vi "insert_block.vi"(8 "error in (no error)":errorcluster, 11 "ImageAssemblerDL090211Frame in":refnum<class "ImageAssemblerDL090211Frame.lvclass">) -> (0 "error out":errorcluster, 3 "ImageAssemblerDL090211Frame out":refnum<class "ImageAssemblerDL090211Frame.lvclass">)   [LabVIEW 2010, in "ImageAssemblerDL090211Frame.lvclass"]
uses:
  ImageAssemblerDL090211Frame.lvclass
  ImageAssemblerDL090211Frame.lvclass/ImageAssemblerDL090211Frame.ctl
  common/classes/Image/Image/Image.lvclass
  common/classes/Image/Image/insert_mode_enum.ctl
  ImagingMode/GenericImagingMode/GenericImagingMode/trigger_enum.ctl
  ImagingMode/GenericImagingMode/GenericImagingMode/GenericImagingMode.lvclass
  common/classes/GenericComponent/GenericComponent/class_data.vi
  ImageAssemblerDL090211Scaffold/ImageAssemblerDL090211Scaffold/ImageAssemblerDL090211Scaffold.lvclass
  common/classes/GenericComponent/GenericComponent/GenericComponent.lvclass
panel:
  out "raw channels":T1[](array[plugin-control])
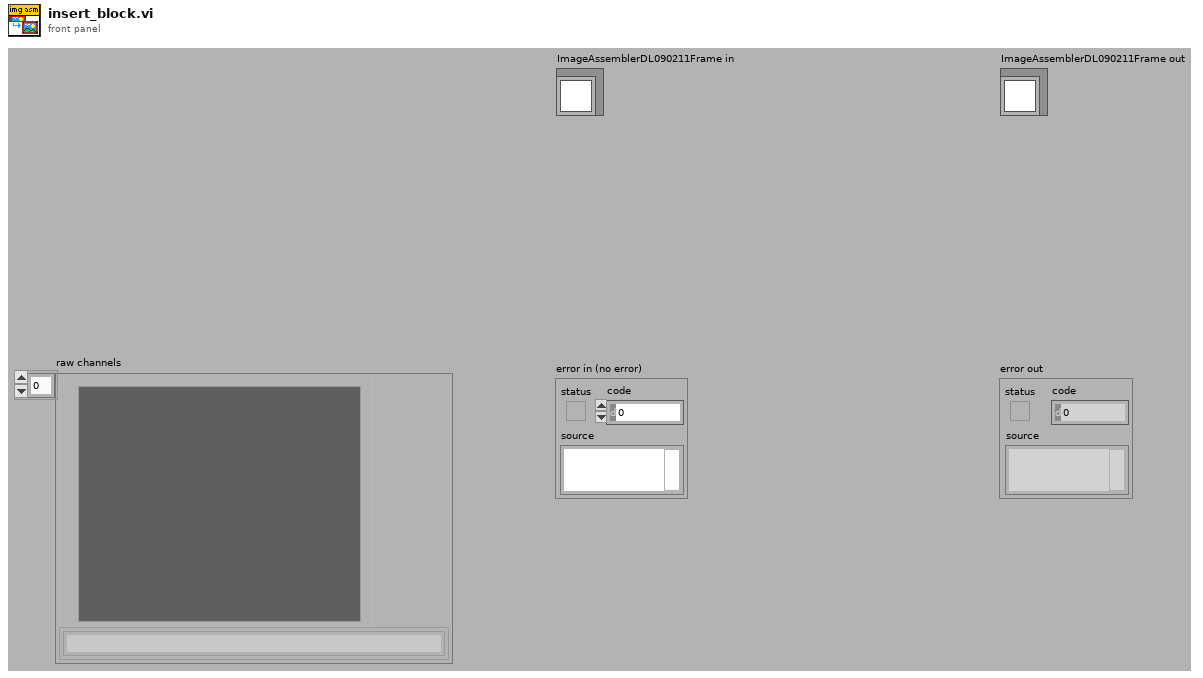
[diagram p1: front panel]
types:
  T1 = typedef "IMAQ Image.ctl" = refnum<image>
  T2 = typedef "Image.lvclass/insert_mode_enum.ctl" = enum16{"replace", "average"}
  T3 = typedef "GenericImagingMode.lvclass/trigger_enum.ctl" = enum16{"NULL", "proceed"}
  T4 = typedef "pixel_raw_data_array.ctl" = dbl[][]
  T5 = typedef "pixel_coordinate_cluster.ctl" = cluster{"x":i32, "y":i32}
  T6 = typedef "Image.lvclass/unit.ctl" = enum16{"um", "s"}
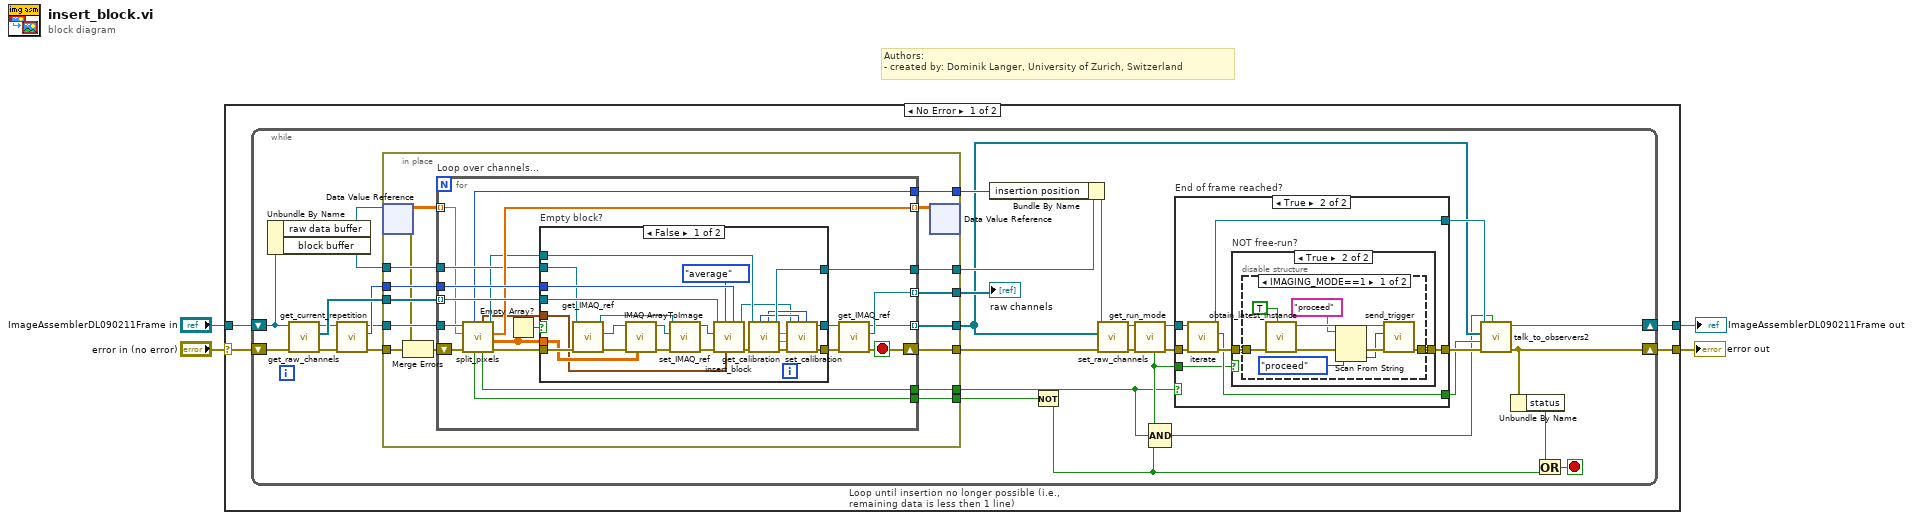
[diagram p0: block diagram]
diagram:
  # "Authors: \n- created by: Dominik Langer, University of Zurich, Switzerland"
  n1 = case shown="No Error" "error in (no error)" {
    selector: "error in (no error)" -> [w8 w129]
    tunnel: [w7 w129] -> w3
    tunnel: [w6 w128] -> w1
    tunnel: "ImageAssemblerDL090211Frame in" -> [w5 w128]
    frame No Error {
      n2 = while "Loop until insertion no longer possible (i.e., remaining data is less then 1 line)" {
        shift-right: [w15] -> w6
        shift-left: w5 -> [w33]
        shift-right: [w16] -> w7
        shift-left: w8 -> [w30]
        stop <- w22 stop-if-true
        n3 = Unbundle By Name(w33) -> ("raw data buffer"=w25:refnum<data-value>, "block buffer"=w35:refnum<class "Image.lvclass">)
        n4 = call-dynamic "get_raw_channels.vi"("error in (no error)"=w30, "DL090211ImageAssemblerScaffold.lvclass in"=w33) -> ("error out"=w37:errorcluster, "raw channels"=w40:refnum<class "Image.lvclass">[], "DL090211ImageAssemblerScaffold.lvclass out"=w36:refnum<class "ImageAssemblerDL090211Frame.lvclass">)  [unwired: 7 out]
        n5 = call "get_current_repetition.vi"("error in (no error)"=w37, "DL090211ImageAssemblerScaffold.lvclass in"=w36) -> ("error out"=w32:errorcluster, "current repetition"=w39:i32, "DL090211ImageAssemblerScaffold.lvclass out"=w38:refnum<class "ImageAssemblerDL090211Frame.lvclass">)  [unwired: 7 out]
        n6 = in-place "In Place Element Structure" {
          in-place-border: w40 -> [w56]
          in-place-border: w39 -> [w55]
          in-place-border: w38 -> [w54]
          in-place-border: [w53] -> w20
          in-place-border: w35 -> [w52]
          in-place-border: [w51] -> w11
          in-place-border: [w50] -> w34
          in-place-border: w32 -> [w45]
          in-place-border: [w49] -> w31
          in-place-border: [w48] -> w13
          in-place-border: [w47] -> w24
          in-place-border: [w42] -> w19
          n7 = in-place-dvr #1(w25) -> (w41:T4, w46:errorcluster)
          n8 = Merge Errors(w46, w45) -> (w44:errorcluster)
          n9 = for "Loop over channels..." {
            shift-right: [w65] -> w49
            shift-left: w44 -> [w71]
            tunnel: w56 -> [w76] mode=indexing
            tunnel: [w62] -> w48 mode=indexing
            tunnel: w55 -> [w77]
            tunnel: [w66] -> w50 mode=indexing
            tunnel: [w75] -> w43 mode=indexing
            tunnel: w54 -> [w70]
            tunnel: [w69] -> w53
            tunnel: w52 -> [w74]
            tunnel: [w72] -> w51
            tunnel: [w73] -> w47
            tunnel: w41 -> [w67] mode=indexing
            tunnel: [w68] -> w42
            stop <- w65 stop-if-true
            n10 = call-dynamic "split_pixels.vi"("error in (no error)"=w71, "pixels in"=w67, "DL090211FrameImageAssembler in"=w70) -> ("error out"=w61:errorcluster, "pixel block"=w58:sgl[][], "for next time"=w75:dbl[], "DL090211FrameImageAssembler out"=w60:refnum<class "ImageAssemblerDL090211Frame.lvclass">, "end of frame reached?"=w72:bool, "insertion coordinate"=w59:T5, "another insertion possible?"=w73:bool, "next inseration coordinate"=w68:u64)  [unwired: 1 out]
            n11 = Empty Array?(array=w58) -> (empty?=w57:bool)
            n12 = case "Empty block?" shown="False" w57 {
              tunnel: w77 -> [w102 _]
              tunnel: w76 -> [w101 w104]
              tunnel: w74 -> [w100 _]
              tunnel: [w99 w105] -> w69
              tunnel: [w98 w103] -> w64
              tunnel: [w97 w104] -> w63
              tunnel: w61 -> [w89 w103]
              tunnel: w58 -> [w88 _]
              tunnel: w60 -> [w85 w105]
              tunnel: w59 -> [w80 _]
              frame False {
                n13 = call-dynamic "get_IMAQ_ref.vi"("error in (no error)"=w89, "Image.lvclass in"=w100) -> ("error out"=w96:errorcluster, "Image"=w95:T1, "Image.lvclass out"=w93:refnum<class "Image.lvclass">)  [unwired: 7 out]
                n14 = call "IMAQ ArrayToImage"("Image Pixels (Float)"=w88, "error in (no error)"=w96, "Image"=w95) -> ("error out"=w94:errorcluster, "Image Out"=w92:T1)  [unwired: 3 in, 4 out]
                n15 = call-dynamic "set_IMAQ_ref.vi"("error in (no error)"=w94, "Image"=w92, "Image.lvclass in"=w93) -> ("error out"=w91:errorcluster, "Image.lvclass out"=w90:refnum<class "Image.lvclass">)  [unwired: 7 out]
                n16 = call-dynamic "insert_block.vi"("repetition"=w102, "start pixel coordinate"=w80, "mode"=insert_mode_enum."average", "error in (no error)"=w91, "block"=w90, "Image in"=w101) -> ("error out"=w79:errorcluster, "Image out"=w78:refnum<class "Image.lvclass">)  [unwired: 4 out]
                n17 = call-dynamic "get_calibration.vi"("error in (no error)"=w79, "ImageAssemblerDL090211Scaffold in"=w85) -> ("error out"=w86:errorcluster, "y"=w83:dbl, "x"=w84:dbl, "ImageAssemblerDL090211Scaffold out"=w99:refnum<class "ImageAssemblerDL090211Frame.lvclass">, "y unit"=w81:T6, "x unit"=w82:T6)  [unwired: 4 in]
                n18 = call "set_calibration.vi"("y unit"=w81, "x unit"=w82, "error in (no error)"=w86, "y"=w83, "x"=w84, "Image in"=w78) -> ("error out"=w98:errorcluster, "Image out"=w97:refnum<class "Image.lvclass">)  [unwired: 4 in]
              }
              frame True {
              }
            }
            n19 = call-dynamic "get_IMAQ_ref.vi"("error in (no error)"=w64, "Image.lvclass in"=w63) -> ("error out"=w65:errorcluster, "Image"=w66:T1, "Image.lvclass out"=w62:refnum<class "Image.lvclass">)  [unwired: 7 out]
          }
          n20 = in-place-dvr #1(w43) -> ()  [unwired: 2 out]
        }
        "raw channels" <- w34
        n21 = Bundle By Name(cluster=w20, "insertion position"=w19) -> (w21:refnum<class "ImageAssemblerDL090211Frame.lvclass">)
        n22 = Not(x=w24) -> (.not. x?=w10:bool)
        n23 = call "set_raw_channels.vi"("error in (no error)"=w31, "raw channels"=w13, "DL090211ImageAssemblerScaffold.lvclass in"=w21) -> ("error out"=w27:errorcluster, "DL090211ImageAssemblerScaffold.lvclass out"=w26:refnum<class "ImageAssemblerDL090211Frame.lvclass">)  [unwired: 7 out]
        n24 = call "get_run_mode.vi"("error in (no error)"=w27, "GenericPlugin in"=w26) -> ("error out"=w29:errorcluster, "GenericPlugin out"=w28:refnum<class "ImageAssemblerDL090211Frame.lvclass">, "is NOT free run?"=w12:bool)  [unwired: 5 in, 2 out]
        n25 = Compound Arithmetic op=AND(w12, w11, w10) -> (w9:bool)
        n26 = case "End of frame reached?" shown="True" w11 {
          tunnel: w29 -> [w106 w114]
          tunnel: w28 -> [w107 w113]
          tunnel: [w107 w109] -> w17
          tunnel: [w106 w111] -> w18
          tunnel: [_ w110] -> w14
          tunnel: w12 -> [_ w108]
          frame False {
          }
          frame True {
            n27 = call-dynamic "iterate.vi"("error in (no error)"=w114, "DL090211ImageAssemblerScaffold in"=w113) -> ("error out"=w112:errorcluster, "finished?"=w110:bool, "DL090211ImageAssemblerScaffold out"=w109:refnum<class "ImageAssemblerDL090211Frame.lvclass">)  [unwired: 7 out]
            n28 = case "NOT free-run?" shown="True" w108 {
              tunnel: w112 -> [w115 w117]
              tunnel: [w115 w116] -> w111
              frame False {
              }
              frame True {
                n29 = disable-structure shown="IMAGING_MODE==1" {
                  disable-tunnel: w117 -> [w125 w127]
                  disable-tunnel: [w126 w127] -> w116
                  frame condition #0 (active) {
                    n30 = call "obtain_latest_instance.vi"("quick, but maybe outdated?"=TRUE, "error in (no error)"=w125) -> ("error out"=w122:errorcluster, "GenericScanMode out"=w124:refnum<class "GenericImagingMode.lvclass">)  [unwired: 8 in]
                    n31 = Scan From String(input string="proceed", error in=w122, default 1=trigger_enum."proceed" ("message")) -> (error out=w121:errorcluster, output 1=w119:T3)  [unwired: 2 in, 2 out]
                    n32 = call-dynamic "send_trigger.vi"("error in (no error)"=w121, "message"=w119, "GenericScanMode in"=w124) -> ("error out"=w126:errorcluster)  [unwired: 8 out]
                  }
                  frame condition #1 {
                  }
                }
              }
            }
          }
        }
        n33 = call-dynamic "talk_to_observers2.vi"("force sending?"=w9, "error in (no error)"=w18, "image finished?"=w14, "image (channels)"=w13, "GenericToplevelComponent in"=w17) -> ("error out"=w16:errorcluster, "GenericToplevelComponent out"=w15:refnum<class "ImageAssemblerDL090211Frame.lvclass">)  [unwired: 5 in]
        n34 = Unbundle By Name(w16) -> ("status"=w23:bool)
        n35 = Or(x=w23, y=w10) -> (x .or. y?=w22:bool)
      }
    }
    frame Error {
    }
  }
  "error out" <- w3
  "ImageAssemblerDL090211Frame out" <- w1
